vi "DEBUG Read Repo.vi"(8 "error in (no error)":errorcluster, 11 "NISE_CEF_Repository in":refnum<class "NISE_CEF_Repository.lvclass">) -> (0 "error out":errorcluster, 3 "String":string)   [LabVIEW 2015, in "Configuration Tool.lvlib"]
uses:
  Configuration Tool.lvlib
  <vilib>/NI/Configuration Framework/Repository/NISE_CEF_Repository.lvclass
  Classes/SequenceRepo/SequenceRepo.lvclass
  Prototype/classes/Sequence/Config/Sequence Config.lvclass
  Prototype/classes/Step/Config/Step Config.lvclass
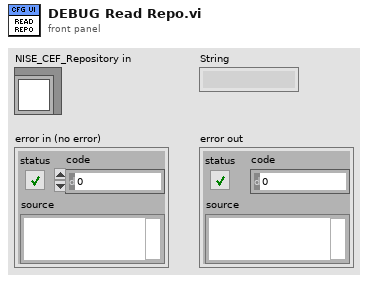
[diagram p1: front panel]
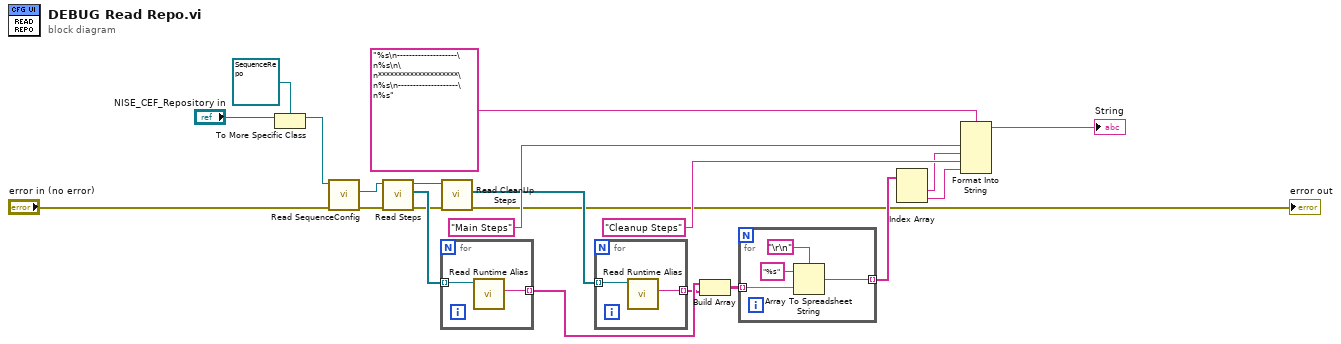
[diagram p0: block diagram]
diagram:
  n1 = To More Specific Class(target class=refnum<class "SequenceRepo.lvclass"> refnum ("SequenceRepo.lvclass"), reference="NISE_CEF_Repository in") -> (specific class reference=w4:refnum<class "SequenceRepo.lvclass">)  [unwired: 1 in, 1 out]
  n2 = call-dynamic "Read SequenceConfig.vi"("error in (no error)"="error in (no error)", "SequenceRepo in"=w4) -> ("error out"=w2:errorcluster, "Sequence Config.lvclass"=w7:refnum<class "Sequence Config.lvclass">)  [unwired: 7 in, 1 out]
  n3 = call-dynamic "Read Steps.vi"("error in (no error)"=w2, "Sequence in"=w7) -> ("error out"=w6:errorcluster, "Steps"=w10:refnum<class "Step Config.lvclass">[], "Sequence out"=w9:refnum<class "Sequence Config.lvclass">)  [unwired: 7 in]
  n4 = for {
    tunnel: w10 -> [w23] mode=indexing
    tunnel: [w22] -> w14 mode=indexing
    n5 = call-dynamic "Read Runtime Alias.vi"("Step Config in"=w23) -> ("Runtime Alias"=w22:string)  [unwired: 8 in, 2 out]
  }
  n6 = call-dynamic "Read CleanUp Steps .vi"("error in (no error)"=w6, "Sequence Config in"=w9) -> ("error out"=→"error out":errorcluster, "CleanUp Steps"=w11:refnum<class "Step Config.lvclass">[])  [unwired: 7 in, 1 out]
  n7 = for {
    tunnel: w11 -> [w25] mode=indexing
    tunnel: [w24] -> w13 mode=indexing
    n8 = call-dynamic "Read Runtime Alias.vi"("Step Config in"=w25) -> ("Runtime Alias"=w24:string)  [unwired: 8 in, 2 out]
  }
  n9 = Build Array(w14, w13) -> (w15:string[][])
  n10 = for {
    tunnel: w15 -> [w27] mode=indexing
    tunnel: [w26] -> w16 mode=indexing
    n11 = Array To Spreadsheet String(delimiter (Tab)="\r\n", array=w27, 3:"%s" ("format string")) -> (spreadsheet string=w26:string)
  }
  n12 = Index Array(array=w16) -> (element #1=w17:string, element #2=w18:string)  [unwired: 2 in]
  n13 = Format Into String(format string="%s\n--------------------\n%s\n\n********************\n%s\n--------------------\n%s", "Main Steps", w17, "Cleanup Steps", w18) -> (resulting string=→"String":string)  [unwired: 2 in, 1 out]
